vi "cRIO Module Information.vi"(8 "error in":errorcluster, 10 "Module":u16, 11 "Refnum in":refnum<k20>) -> (0 "error out":errorcluster, 2 "cRIO Module Information":T1 {"Module Code" format="%.0x"}, 3 "Refnum out":refnum<k20>)   [LabVIEW 2015, in "SMI.lvlib" / "Module.lvclass"]
uses:
  Module.lvclass
  Controls/ModuleInformation.ctl
  <vilib>/Utility/error.llb/Error Cluster From Error Code.vi
  <vilib>/rvi/errors/niLvFpgaAdjustHostInterfaceError.vi
  <vilib>/rvi/interface/nirviReadWriteControl/nirviReadWriteControl.xnode
  <vilib>/ErrorRing/Error Ring.xnode
  NiFpgaLv.dll
  <vilib>/rvi/interface/Simulation/niFpgaSimulationCallBeginRW.vi
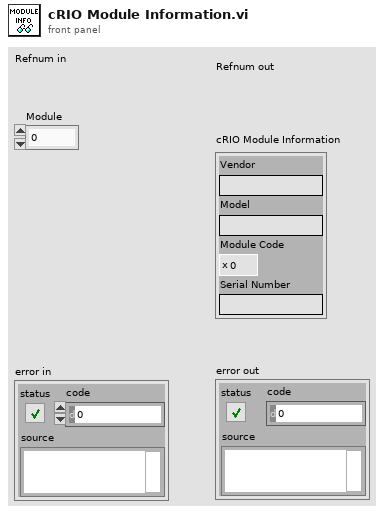
[diagram p1: front panel]
types:
  T1 = typedef "SMI.lvlib/Module.lvclass/ModuleInformation.ctl" = cluster{"Vendor":string, "Model":string, "Module Code":u32, "Serial Number":string}
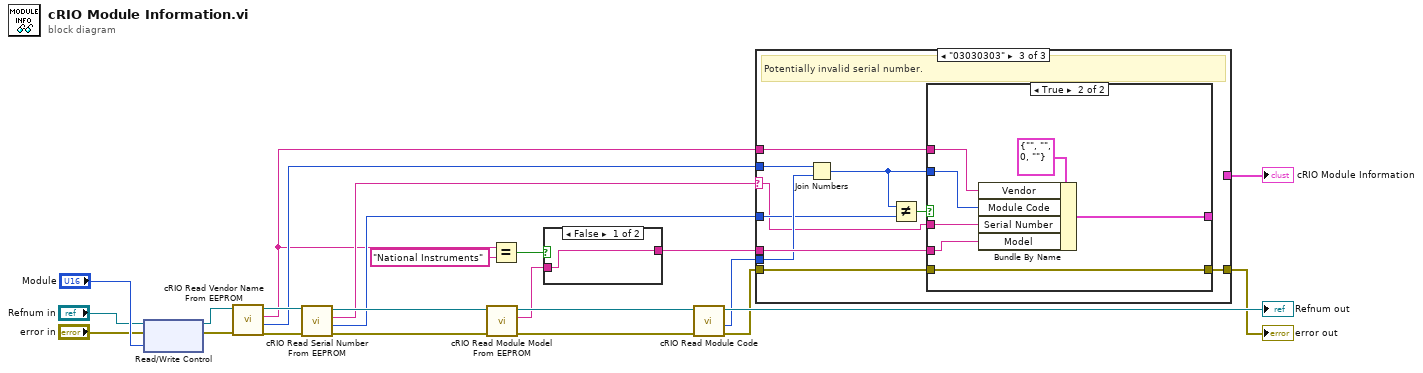
[diagram p0: block diagram]
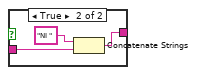
[diagram p2: hidden frame]
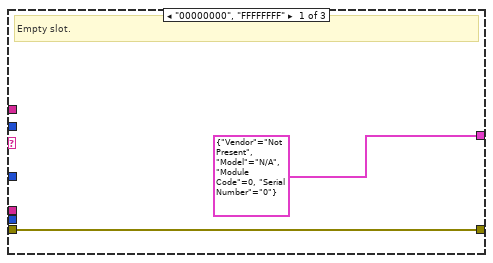
[diagram p3: hidden frame]
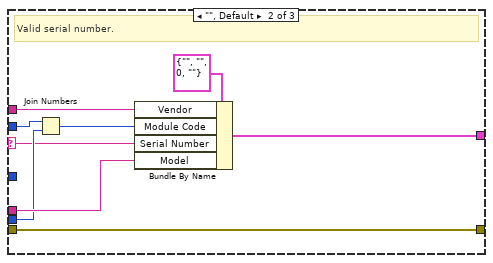
[diagram p4: hidden frame]
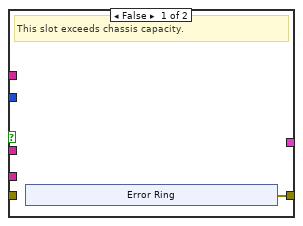
[diagram p5: hidden frame]
diagram:
  n1 = xnode "Read/Write Control"("FPGA VI Reference In"="Refnum in", "error in"="error in", "Module"="Module") -> ("FPGA VI Reference Out"=w18:refnum<k20>, "error out"=w19:errorcluster)
  n2 = call "cRIO Read Vendor Name From EEPROM.vi"("error in"=w19, "Refnum in"=w18) -> ("error out"=w21:errorcluster, "Vendor ID"=w11:u16, "Vendor Name"=w8:string, "Refnum out"=w22:refnum<k20>)  [unwired: 6 in]
  n3 = call "cRIO Read Serial Number From EEPROM.vi"("error in"=w21, "Refnum in"=w22) -> ("error out"=w24:errorcluster, "Serial Number"=w9:u32, "Serial Number String"=w15:string, "Refnum out"=w23:refnum<k20>)  [unwired: 6 in]
  n4 = call "cRIO Read Module Model From EEPROM.vi"("error in"=w24, "Refnum in"=w23) -> ("error out"=w14:errorcluster, "Module Model"=w5:string, "Refnum out"=w13:refnum<k20>)  [unwired: 7 in]
  n5 = Equal?(x=w8, y="National Instruments") -> (x = y?=w6:bool)
  n6 = case shown="False" w6 {
    tunnel: w5 -> [w25 w27]
    tunnel: [w25 w26] -> w4
    frame False {
    }
    frame True {
      n7 = Concatenate Strings("NI " ("string"), w27) -> (w26:string)
    }
  }
  n8 = call "cRIO Read Module Code.vi"("error in"=w14, "Refnum in"=w13) -> ("error out"=w3:errorcluster, "Module ID"=w10:u16, "Refnum out"=→"Refnum out":refnum<k20>)  [unwired: 6 in, 1 out]
  n9 = case shown="\"03030303\"" w15 {
    selector: w15 -> [_ w31 w40]
    tunnel: w8 -> [_ w39 w49]
    tunnel: w4 -> [_ w38 w48]
    tunnel: [T1 {"Vendor"="Not Present", "Model"="N/A", "Module Code"=0, "Serial Number"="0"} ("cRIO Module Information") w37 _] -> w1
    tunnel: w10 -> [_ w36 w47]
    tunnel: w11 -> [_ w35 w46]
    tunnel: w9 -> [_ _ w41]
    tunnel: w3 -> [w30 w32 w44]
    tunnel: [w30 w32 w43] -> w2
    frame "00000000", "FFFFFFFF" {
      # "Empty slot."
    }
    frame "", Default {
      # "Valid serial number."
      n10 = Join Numbers(hi=w35, lo=w36) -> ((hi.lo)=w33:u32)
      n11 = Bundle By Name(cluster=T1 {"Vendor"="", "Model"="", "Module Code"=0, "Serial Number"=""} ("Module Information"), "Vendor"=w39, "Module Code"=w33, "Serial Number"=w31, "Model"=w38) -> (w37:T1)
    }
    frame "03030303" {
      # "Potentially invalid serial number."
      n12 = Join Numbers(hi=w46, lo=w47) -> ((hi.lo)=w42:u32)
      n13 = Not Equal?(x=w42, y=w41) -> (x != y?=w45:bool)
      n14 = case shown="True" w45 {
        tunnel: w49 -> [_ w61]
        tunnel: w48 -> [_ w60]
        tunnel: [_ w59] -> _
        tunnel: w40 -> [_ w58]
        tunnel: w42 -> [_ w56]
        tunnel: w44 -> [_ w55]
        tunnel: [w50 w55] -> w43
        frame False {
          # "This slot exceeds chassis capacity."
          n15 = xnode "Error Ring"() -> ("error out"=w50:errorcluster)
        }
        frame True {
          n16 = Bundle By Name(cluster=T1 {"Vendor"="", "Model"="", "Module Code"=0, "Serial Number"=""} ("Module Information"), "Vendor"=w61, "Module Code"=w56, "Serial Number"=w58, "Model"=w60) -> (w59:T1)
        }
      }
    }
  }
  "error out" <- w2
  "cRIO Module Information" <- w1
